vi "GageAvgSpec_test_och_loop.vi"() -> ()   [LabVIEW 2016]
uses:
  <vilib>/express/express analysis/Spectral/XNode/ExpressSpectralMeasurementsBlockNode.xnode
  <vilib>/express/express analysis/Spectral/Block/exnSpectralBlock spectral measurements power poly.vi
  <vilib>/express/express analysis/Spectral/Block/exnSpectralBlock spectral measurements power WFM.vi
  <vilib>/Utility/file.llb/Write To Spreadsheet File (DBL).vi
panel:
  in  "Continuous":bool=TRUE
  out "루프 사이의 time interval":dbl
  out "100 세트 저장완료 5":bool
  in  "데이터 저장 시작 5":bool
  out "Spec(ch0) 6":cluster{"f0":dbl, "df":dbl, "magnitude":dbl[]}(graph)
  out "Spec(ch2) 6":cluster{"f0":dbl, "df":dbl, "magnitude":dbl[]}(graph)
  out "Spec(ch3) 6":cluster{"f0":dbl, "df":dbl, "magnitude":dbl[]}(graph)
  in  "Start 6":i32
  in  "Points 6":u32=4096
  in  "Averages 7":u32=1 min=1 step=1
  in  "Channels 4":T1(array[cluster])=[{"Coupling"=0, "Differential Input"=FALSE, "Direct-to-ADC"=FALSE, "Range"=2000, "Impedance"=50, "Filter"=0}] {"Impedance" min=50 max=1000000 step=999950; "Coupling" items=["DC", "AC"]}
  in  "Trigger 3":T2={"Slope"=0, "Level"=0, "Source"=0, "External Range"=2000, "External Coupling"=0, "External"=FALSE, "Disable"=FALSE, "External Impedance"=1} {"External Impedance" items=["50 Ohm", "HiZ"]; "External Coupling" items=["DC", "AC"]; "External Range" min=2000 max=10000 step=8000; "Slope" items=["Rising", "Falling"]; "Level" min=-100 max=100; "Source" min=0 max=64 step=1}
  in  "Acquisition 4":T3={"Sample Rate"=50000000.0, "Mode"=2, "Depth"=8192.0, "Segment Size"=8192.0, "Trigger Timeout"=1000000.0, "Trigger Holdoff"=0.0, "Trigger Delay"=0.0, "Clock mode"=enum."Internal"} {"Segment Size" min=256.0 step=128.0; "Trigger Holdoff" min=0.0 step=128.0; "Trigger Delay" min=0.0 step=128.0; "Depth" min=256.0 step=128.0; "Mode" items=["Single", "Dual", "Quad", "Octal"]}
  in  "Averages 3":u32=1 min=1 step=1
  in  "Averaging Method 3":bool
  out "Progress 5":string
  in  "stop 5":bool
  out "System Count":i32
  out "Sample Bits 2":i32
  out "Board Count 2":i32
  out "Channel Count 2":i32
  out "Trigger Count 2":i32
  out "System Name 2":string
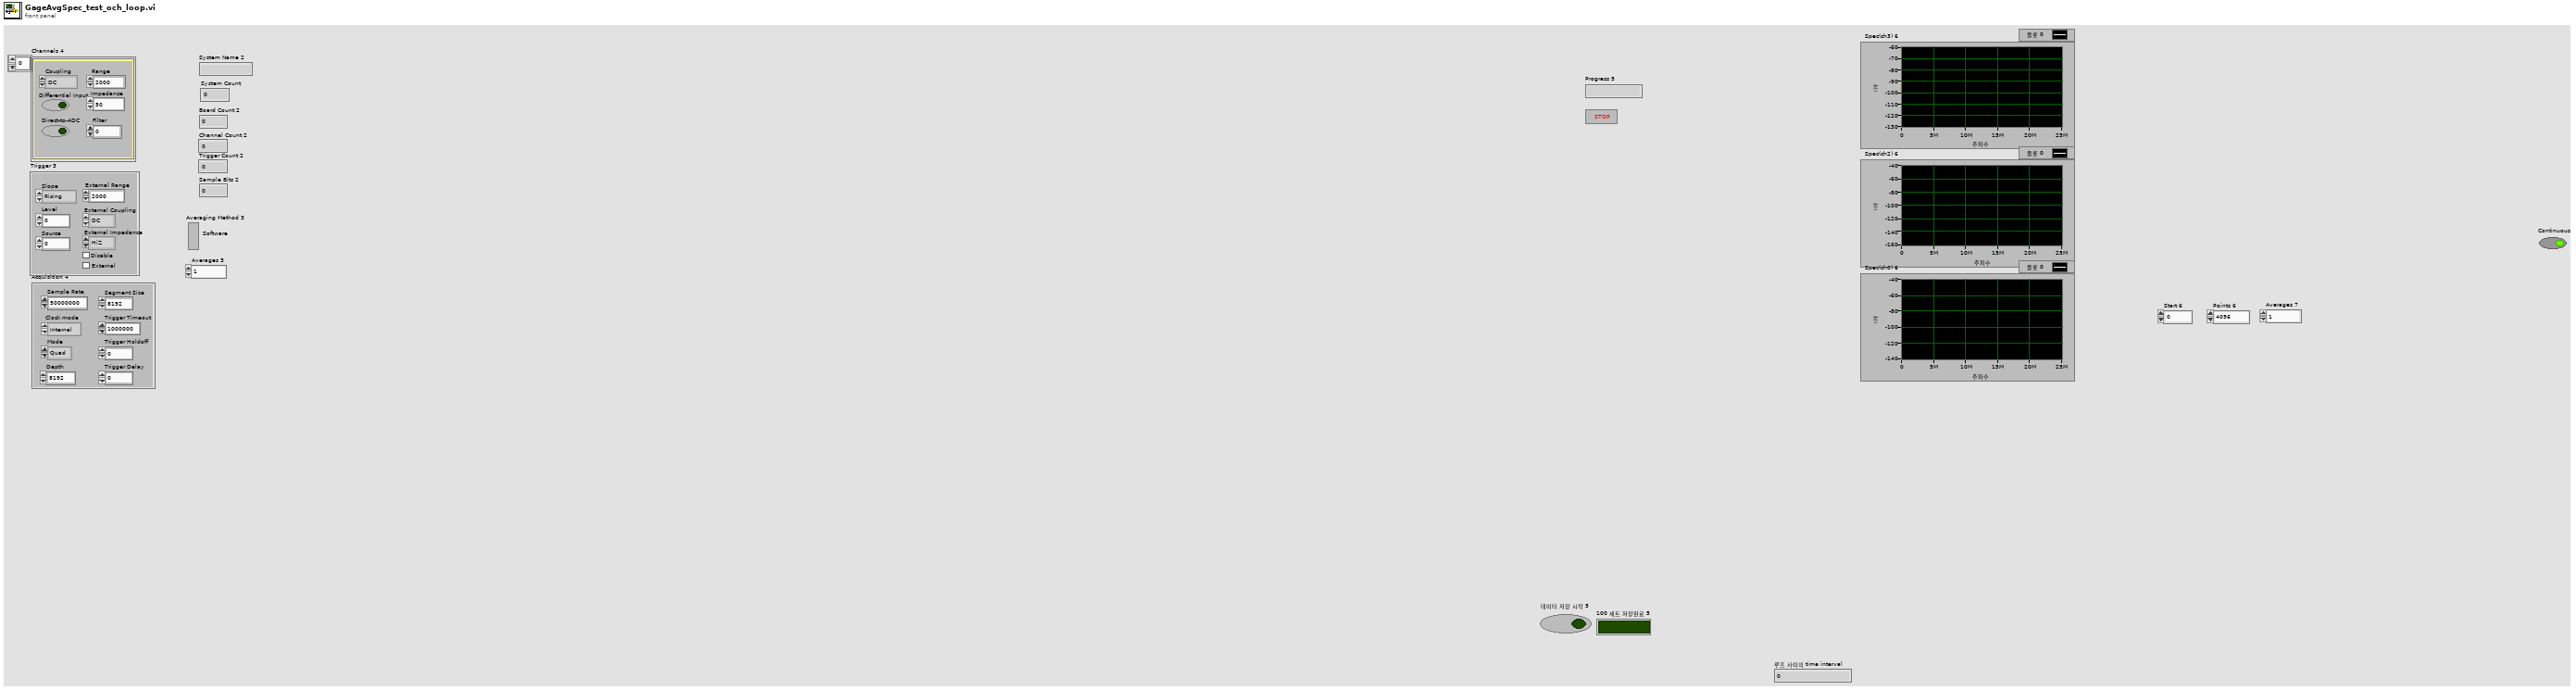
[diagram p1: front panel]
types:
  T1 = cluster{"Coupling":u16, "Differential Input":bool, "Direct-to-ADC":bool, "Range":u32, "Impedance":u32, "Filter":i32}[]
  T2 = cluster{"Slope":u16, "Level":i32, "Source":i32, "External Range":u32, "External Coupling":u16, "External":bool, "Disable":bool, "External Impedance":u16}
  T3 = cluster{"Sample Rate":dbl, "Mode":u16, "Depth":dbl, "Segment Size":dbl, "Trigger Timeout":dbl, "Trigger Holdoff":dbl, "Trigger Delay":dbl, "Clock mode":enum16{"Internal", "External", "Reference"}}
  T4 = cluster{"Handle":u32, "Sample size":u32, "Resolution":i32, "Offset":i32, "Channels":u32, "Boards":u32}
  T5 = cluster{"averaging mode":u16, "weighting mode":u16, "number of averages":u32}
  T6 = cluster{"dB On (F)":bool, "unwrap phase (F)":bool, "convert to degree (F)":bool}
  T7 = cluster{string, "Differential Input":bool, "Direct-to-ADC":bool, "Range":u32, "Impedance":u32, i32, "Filter":i32}
  T8 = cluster{"RingText.Text":string, "Level":i32, "Source":i32, "External Range":u32, "RingText.Text":string, "External":bool, "Disable":bool, "RingText.Text":string}
  T9 = cluster{"RingText.Text":string, "Level":i32, "Source":i32, "External Range":u32, "RingText.Text":string, "External":bool, "Disable":bool, "RingText.Text":string}[]
  T10 = cluster{"Handle":u32, "Sample Size":u32, "Resolution":i32, "Offset":i32, "Channels":u32, "Boards":u32}
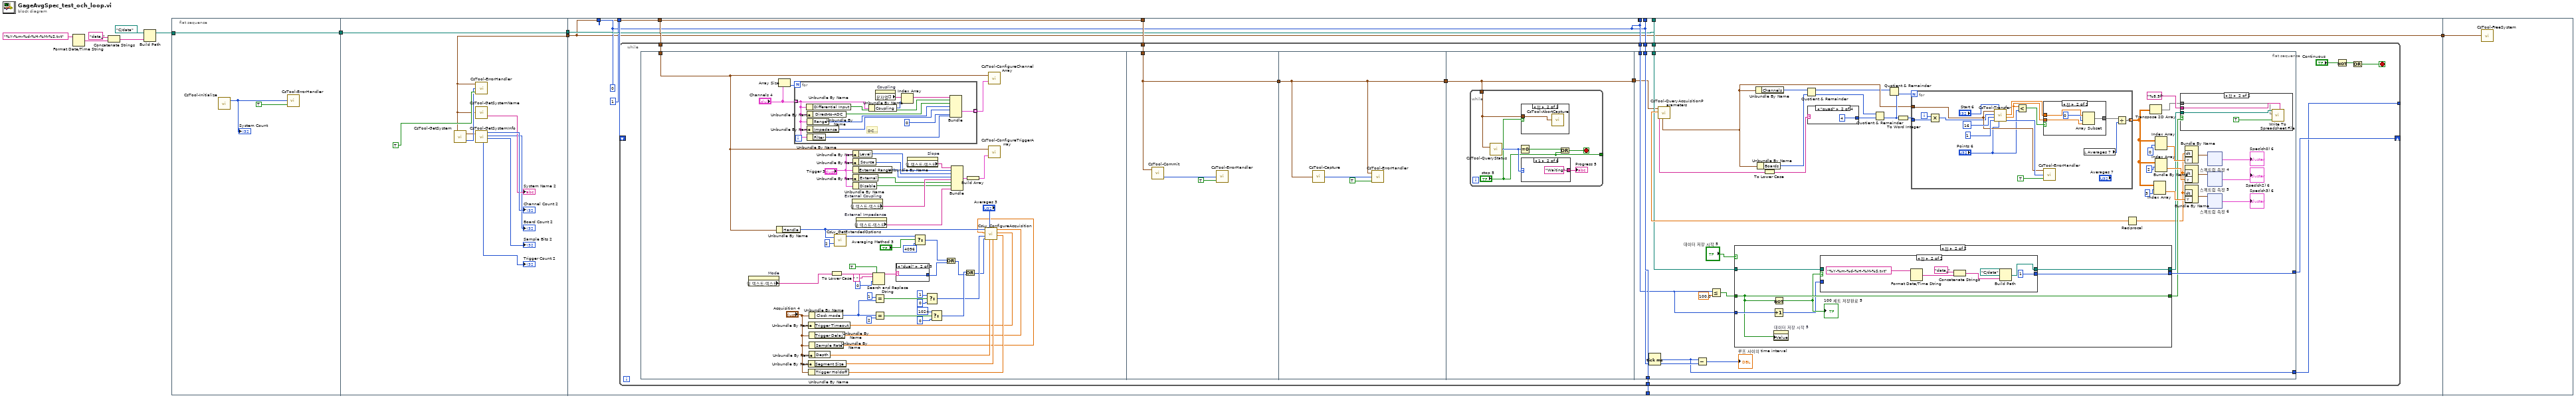
[diagram p0: block diagram]
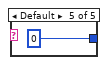
[diagram p5: hidden frame]
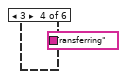
[diagram p9: hidden frame]
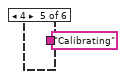
[diagram p10: hidden frame]
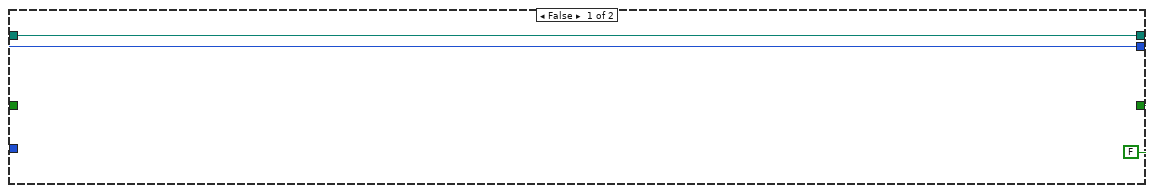
[diagram p13: hidden frame]
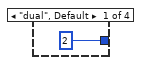
[diagram p15: hidden frame]
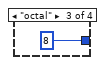
[diagram p16: hidden frame]
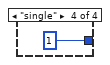
[diagram p17: hidden frame]
diagram:
  n1 = Format Date/Time String(time format string (%c)="%Y-%m-%d-%H-%M-%S.txt" ("시간 포맷 문자열 (%c)")) -> (date/time string=w13:string)  [unwired: 2 in]
  n2 = Concatenate Strings "Concatenate Strings"("data_", w13) -> (w12:string)
  n3 = Build Path(base path=path "C:/data", name or relative path=w12) -> (appended path=w9:path)
  n4 = flat-sequence {
    tunnel: w9 -> [w18]
    tunnel: [w18] -> w10
    tunnel: [w22] -> w17
    tunnel: w10 -> [w21]
    tunnel: [w21] -> w8
    tunnel: w17 -> [w30]
    tunnel: [w30] -> w11
    tunnel: w8 -> [w33]
    tunnel: [w31] -> _
    tunnel: [w30] -> w7
    tunnel: [w31] -> w6
    tunnel: [w31] -> w5
    tunnel: [w31] -> _
    tunnel: [w31] -> w4
    tunnel: [w33] -> w3
    tunnel: [1] -> w2
    tunnel: [w31] -> _
    tunnel: [w30] -> w1
    tunnel: w1 -> [w34]
    frame #0 {
      n5 = call <userlib>:"CsTool-Initialize.vi"() -> ("Number Of Systems"=w20:i32)  [unwired: 1 out]
      "System Count" <- w20
      n6 = call <userlib>:"CsTool-ErrorHandler.vi"("StopOnError (true)"=TRUE, "Error Code"=w20) -> ()  [unwired: 1 in, 1 out]
    }
    frame #1 {
      n7 = call <userlib>:"CsTool-GetSystem.vi"() -> ("Error Code"=w23:i32, "Handle Cluster"=w22:T4)  [unwired: 4 in]
      n8 = call <userlib>:"CsTool-ErrorHandler.vi"("StopOnError (true)"=TRUE, "Error Code"=w23, "Handle Cluster"=w22) -> ()  [unwired: 1 out]
      n9 = call <userlib>:"CsTool-GetSystemName.vi"("Handle Cluster"=w22) -> ("System Name"=→"System Name 2":string)  [unwired: 1 out]
      n10 = call <userlib>:"CsTool-GetSystemInfo.vi"("Handle Cluster"=w22) -> ("Number Of Triggers"=→"Trigger Count 2":u32, "Number Of Channels"=→"Channel Count 2":u32, "Number Of Boards"=→"Board Count 2":u32, "Sample Bits"=→"Sample Bits 2":u32)  [unwired: 3 out]
    }
    frame #2 {
      w31 = 0
    }
    frame #3 {
      n11 = call <userlib>:"CsTool-FreeSystem.vi"("Handle Cluster"=w34) -> ()  [unwired: 1 out]
    }
  }
  n12 = while {
    tunnel: w11 -> [w47]
    tunnel: w7 -> [w45]
    tunnel: w6 -> [w43]
    tunnel: w5 -> [w42]
    tunnel: w4 -> [w41]
    tunnel: w3 -> [w40]
    shift-right: [w36] -> _
    shift-left: w2 -> [_]
    tunnel: [w35] -> _
    stop <- w37 stop-if-true
    n13 = flat-sequence {
      tunnel: w47 -> [w49]
      tunnel: [w113] -> w46
      tunnel: w45 -> [w113]
      tunnel: [w116] -> w48
      tunnel: w46 -> [w116]
      tunnel: w48 -> [w119]
      tunnel: [w119] -> w44
      tunnel: w44 -> [w133]
      tunnel: w43 -> [_]
      tunnel: w42 -> [w144]
      tunnel: [w143] -> w35
      tunnel: [w142] -> w36
      tunnel: w41 -> [w137]
      tunnel: w40 -> [w136]
      frame #0 {
        n14 = property on="Mode" class="Ring (엄격한)"() -> ("링 텍스트.텍스트"=w53:string)  [unwired: 2 in, 2 out]
        n15 = Unbundle By Name(w49) -> ("Handle"=w56:u32)
        n16 = Array Size(array="Channels 4") -> (size(s)=w95:i32)
        n17 = for {
          N: w95 -> [_]
          tunnel: "Channels 4" -> [w100] mode=indexing
          tunnel: [w104] -> w96 mode=indexing
          # "DC Offset"
          n18 = Unbundle By Name(w100) -> ("Differential Input"=w107:bool)
          n19 = Unbundle By Name(w100) -> ("Direct-to-ADC"=w106:bool)
          n20 = Unbundle By Name(w100) -> ("Range"=w97:u32)
          n21 = Unbundle By Name(w100) -> ("Impedance"=w105:u32)
          n22 = Unbundle By Name(w100) -> ("Filter"=w99:i32)
          n23 = Unbundle By Name(w100) -> ("Coupling"=w102:u16)
          n24 = property on="Coupling" class="Ring (엄격한)"() -> ("문자열[]"=w103:string[])  [unwired: 2 in, 2 out]
          n25 = Index Array(array=w103, index=w102) -> (element=w101:string)
          n26 = Bundle(w101, "Differential Input"=w107, "Direct-to-ADC"=w106, "Range"=w97, "Impedance"=w105, 0, "Filter"=w99) -> (w104:T7)  [unwired: 1 in]
        }
        n27 = Unbundle By Name("Acquisition 4") -> ("Trigger Timeout"=w65:dbl)
        n28 = Unbundle By Name("Acquisition 4") -> ("Segment Size"=w80:dbl)
        n29 = Unbundle By Name("Acquisition 4") -> ("Trigger Holdoff"=w81:dbl)
        n30 = Unbundle By Name("Acquisition 4") -> ("Clock mode"=w76:enum16{"Internal", "External", "Reference"})
        n31 = Unbundle By Name("Acquisition 4") -> ("Trigger Delay"=w66:dbl)
        n32 = Unbundle By Name("Acquisition 4") -> ("Sample Rate"=w50:dbl)
        n33 = Unbundle By Name("Acquisition 4") -> ("Depth"=w79:dbl)
        n34 = To Lower Case(string=w53) -> ()  [unwired: 1 out]
        n35 = call <userlib>:"CsLv_GetExtendedOptions.vi"("Handle"=w56, "Option"=2) -> ("User Mode"=w58:u32)  [unwired: 2 out]
        n36 = property on="External Coupling" class="Ring (엄격한)"() -> ("링 텍스트.텍스트"=w91:string)  [unwired: 2 in, 2 out]
        n37 = Unbundle By Name("Trigger 3") -> ("Level"=w83:i32)
        n38 = Unbundle By Name("Trigger 3") -> ("Source"=w86:i32)
        n39 = Unbundle By Name("Trigger 3") -> ("External Range"=w84:u32)
        n40 = Unbundle By Name("Trigger 3") -> ("External"=w87:bool)
        n41 = Unbundle By Name("Trigger 3") -> ("Disable"=w88:bool)
        n42 = property on="External Impedance" class="Ring (엄격한)"() -> ("링 텍스트.텍스트"=w92:string)  [unwired: 2 in, 2 out]
        n43 = Search and Replace String(replace all?=TRUE, input string=w53, search string=" ", offset=0) -> (result string=w54:string)  [unwired: 4 in, 3 out]
        n44 = Equal?(x=1, y=w76) -> (x = y?=w72:bool)
        n45 = Equal?(x=w76, y=2) -> (x = y?=w74:bool)
        n46 = case shown="\"dual\"" w54 {
          tunnel: [1 2 4 8 0] -> w62
          frame "single" {
          }
          frame "dual" {
          }
          frame "quad" {
          }
          frame "octal" {
          }
          frame Default {
          }
        }
        n47 = property on="Slope" class="Ring (엄격한)"() -> ("링 텍스트.텍스트"=w90:string)  [unwired: 2 in, 2 out]
        n48 = Select(t=w58, s="Averaging Method 3", f=4096) -> (s? t:f=w61:u32)
        n49 = Select(t=u32 1, s=w72, f=u32 0) -> (s? t:f=w77:u32)
        n50 = Select(t=1024, s=w74, f=0) -> (s? t:f=w78:i32)
        n51 = Or(x=w61, y=w62) -> (x .or. y?=w60:u32)
        n52 = Bundle("RingText.Text"=w90, "Level"=w83, "Source"=w86, "External Range"=w84, "RingText.Text"=w91, "External"=w87, "Disable"=w88, "RingText.Text"=w92) -> (w85:T8)  [unwired: 1 in]
        n53 = Or(x=w78, y=w60) -> (x .or. y?=w63:u32)
        n54 = Build Array(w85) -> (w93:T9)
        n55 = call <userlib>:"CsLv_ConfigureAcquisition.vi"("Trigger Holdoff (0)"=w81, "Trigger Timeout (10000000)"=w65, "Trigger Delay (0)"=w66, "Segment Size (8192)"=w80, "Depth (8192)"=w79, "Segment Count (1)"="Averages 3", "Mode (2)"=w63, "External Clock (0)"=w77, "Sample Rate (100000000)"=w50, "Handle"=w56) -> ()  [unwired: 1 in, 1 out]
        n56 = call <userlib>:"CsTool-ConfigureChannelArray.vi"("Channels"=w96, "Handle Cluster"=w49) -> ()  [unwired: 1 out]
        n57 = call <userlib>:"CsTool-ConfigureTriggerArray.vi"("Triggers"=w93, "Handle Cluster"=w49) -> ()  [unwired: 1 out]
      }
      frame #1 {
        n58 = call <userlib>:"CsTool-Commit.vi"("Handle Cluster"=w113) -> ("Error Code"=w115:i32)  [unwired: 2 in, 1 out]
        n59 = call <userlib>:"CsTool-ErrorHandler.vi"("StopOnError (true)"=TRUE, "Error Code"=w115) -> ()  [unwired: 1 in, 1 out]
      }
      frame #2 {
        n60 = call <userlib>:"CsTool-Capture.vi"("Handle Cluster"=w116) -> ("Error Code"=w118:i32)
        n61 = call <userlib>:"CsTool-ErrorHandler.vi"("StopOnError (true)"=TRUE, "Error Code"=w118, "Handle Cluster"=w116) -> ()  [unwired: 1 out]
      }
      frame #3 {
        n62 = while {
          tunnel: ["stop 5"] -> _
          tunnel: w119 -> [w120]
          stop <- w122 stop-if-true
          n63 = call <userlib>:"CsTool-QueryStatus.vi"("Handle Cluster"=w120) -> ("Status"=w125:i32)
          n64 = Equal To 0?(x=w125) -> (x = 0?=w123:bool)
          n65 = case shown="참" "stop 5" {
            tunnel: w120 -> [_ w126]
            frame False {
            }
            frame True {
              n66 = call <userlib>:"CsTool-AbortCapture.vi"("Handle Cluster"=w126) -> ()  [unwired: 1 out]
            }
          }
          n67 = case shown="1" w125 {
            tunnel: ["Ready" "Waiting" "Triggered" "Transferring" "Calibrating" " "] -> w124
            frame 0 {
            }
            frame 1 {
            }
            frame 2 {
            }
            frame 3 {
            }
            frame 4 {
            }
            frame 5, Default {
            }
          }
          "Progress 5" <- w124
          n68 = Or(x=w123, y="stop 5") -> (x .or. y?=w122:bool)
        }
      }
      frame #4 {
        n69 = Tick Count (ms)() -> (millisecond timer value=w143:u32)
        n70 = call <userlib>:"CsTool-QueryAcquisitionParameters.vi"("Handle Cluster"=w133) -> ("Output Handle Cluster"=w150:T10, "Mode"=w151:string, "Sample Rate"=w149:dbl)  [unwired: 8 out]
        n71 = Subtract(x=w143, y=w144) -> (x-y=→"루프 사이의 time interval":u32)
        n72 = Less Or Equal?(x=w137, y=100.0) -> (x <= y?=w148:bool)
        n73 = case shown="참" "데이터 저장 시작 5" {
          tunnel: [FALSE w185] -> w141
          tunnel: w148 -> [_ w185]
          tunnel: [w179 w182] -> w142
          tunnel: w137 -> [w179 w186]
          tunnel: w136 -> [w177 w181]
          tunnel: [w177 w180] -> w140
          frame False {
          }
          frame True {
            n74 = Increment(x=w186) -> (x+1=w183:i32)
            n75 = Not(x=w185) -> (.not. x?=w184:bool)
            "100 세트 저장완료 5" <- w184
            n76 = property on="데이터 저장 시작 5" class="Bool (엄격한)"("Value"=w185) -> ()  [unwired: 2 in, 2 out]
            n77 = case shown="참" w184 {
              tunnel: [w188 1] -> w182
              tunnel: w183 -> [w188 _]
              tunnel: w181 -> [w187 _]
              tunnel: [w187 w189] -> w180
              frame False {
              }
              frame True {
                n78 = Format Date/Time String(time format string (%c)="%Y-%m-%d-%H-%M-%S.txt" ("시간 포맷 문자열 (%c)")) -> (date/time string=w191:string)  [unwired: 2 in]
                n79 = Concatenate Strings("data_", w191) -> (w190:string)
                n80 = Build Path(base path=path "C:/data", name or relative path=w190) -> (appended path=w189:path)
              }
            }
          }
        }
        n81 = Unbundle By Name(w150) -> ("Channels"=w167:u32)
        n82 = Unbundle By Name(w150) -> ("Boards"=w170:u32)
        n83 = To Lower Case(string=w151) -> (all lower case string=w171:string)
        n84 = Quotient & Remainder(x=w167, y=w170) -> (x-y*floor(x/y)=w134:u32, floor(x/y)=w169:u32)
        n85 = case shown="\"quad\"" w171 {
          tunnel: [2 4 8 1] -> w168
          frame "dual", Default {
          }
          frame "quad" {
          }
          frame "octal" {
          }
          frame "single" {
          }
        }
        n86 = Quotient & Remainder(x=w169, y=w168) -> (floor(x/y)=w166:u32)  [unwired: 1 out]
        n87 = Quotient & Remainder(x=w134, y=w166) -> (floor(x/y)=w165:u32)  [unwired: 1 out]
        n88 = To Word Integer(number=w166) -> (16bit integer=w172:i16)
        n89 = for {
          N: w165 -> [_]
          tunnel: w150 -> [w232]
          tunnel: [w228] -> w152 mode=indexing
          tunnel: w172 -> [w233]
          i -> [w241]
          n90 = Multiply(x=w241, y=w233) -> (x*y=w231:i32)
          n91 = call <userlib>:"CsTool-Transfer.vi"("Length (4096)"="Points 6", "Start (0)"="Start 6", "Segment (1)"=1, "Mode (0)"=16, "Channel (0)"=w231, "Handle Cluster"=w232) -> ("Error Code"=w236:i32, "Actual Length"=w239:dbl, "Data in Volts"=w229:dbl[])  [unwired: 1 out]
          n92 = Less?(x=w239, y="Points 6") -> (x < y?=w242:bool)
          n93 = case shown="참" w242 {
            tunnel: w229 -> [w243 w247]
            tunnel: w239 -> [_ w245]
            tunnel: [w243 w244] -> w230
            frame False {
            }
            frame True {
              n94 = Array Subset(array=w247, index=0, length=w245) -> (w244:dbl[])
            }
          }
          n95 = call <userlib>:"CsTool-ErrorHandler.vi"("StopOnError (true)"=TRUE, "Error Code"=w236, "Handle Cluster"=w232) -> ()  [unwired: 1 out]
          n96 = local read "Averages 7"() -> (w234:u32)
          n97 = Divide(x=w230, y=w234) -> (x/y=w228:dbl[])
        }
        n98 = Reciprocal(x=w149) -> (1/x=w135:dbl)
        n99 = Transpose 2D Array(2D array=w152) -> (transposed array=w138:dbl[][])
        n100 = Index Array(array=w152, index (row)=3 ("인덱스 (행)")) -> (element=w159:dbl[])  [unwired: 1 in]
        n101 = Index Array(array=w152, index (row)=0 ("인덱스 (행)")) -> (element=w163:dbl[])  [unwired: 1 in]
        n102 = Index Array(array=w152, index (row)=2 ("인덱스 (행)")) -> (element=w161:dbl[])  [unwired: 1 in]
        n103 = case shown="참" w141 {
          tunnel: w140 -> [_ w176]
          tunnel: "%8.5f" ("format (%.3f)") -> [_ w174]
          tunnel: w138 -> [_ w173]
          frame False {
          }
          frame True {
            n104 = call-poly <vilib>:"Write To Spreadsheet File.vi"("format (%.3f)"=w174, "append to file? (new file:F)"=TRUE, "2D data"=w173, "file path (dialog if empty)"=w176) -> ()  [unwired: 4 in, 1 out]
          }
        }
        n105 = Bundle By Name("dt"=w135, "Y"=w163) -> (w164:waveform(dbl))  [unwired: 1 in]
        n106 = Bundle By Name("dt"=w135, "Y"=w161) -> (w162:waveform(dbl))  [unwired: 1 in]
        n107 = Bundle By Name("dt"=w135, "Y"=w159) -> (w160:waveform(dbl))  [unwired: 1 in]
        n108 = xnode "스펙트럼 측정 4"("신호"=w164) -> ("파워 스펙트럼"=→"Spec(ch0) 6":cluster{"f0":dbl, "df":dbl, "magnitude":dbl[]})  [unwired: 1 in, 1 out]
        n109 = xnode "스펙트럼 측정 5"("신호"=w162) -> ("파워 스펙트럼"=→"Spec(ch2) 6":cluster{"f0":dbl, "df":dbl, "magnitude":dbl[]})  [unwired: 1 in, 1 out]
        n110 = xnode "스펙트럼 측정 6"("신호"=w160) -> ("파워 스펙트럼"=→"Spec(ch3) 6":cluster{"f0":dbl, "df":dbl, "magnitude":dbl[]})  [unwired: 1 in, 1 out]
      }
    }
    n111 = Not(x="Continuous") -> (.not. x?=w39:bool)
    n112 = Or(x=w39) -> (x .or. y?=w37:bool)  [unwired: 1 in]
  }
